vi "MC AOTF Engine.vi"(0 "Notifier Name":string, 11 "Ports (Unused)":string[](array[string])) -> ()   [LabVIEW 2016]
uses:
  AOTF Controls/AOTF Notifier Element.ctl
  AOTF Controls/AOTF Actions.ctl
  AOTF Controls/AOTF Lines Lines Control.ctl
  <vilib>/ULx/Create Channel.llb/ULx Create Channel (DO-Digital Output).vi
  <vilib>/ULx/Write.llb/ULx Write (Digital Bool 1Line 1Point).vi
  <vilib>/ULx/Create Channel.llb/ULx Create Channel (AO-Voltage-Basic).vi
  <vilib>/ULx/Write.llb/ULx Write (Analog 1D DBL 1Chan 1Samp).vi
panel:
  in  "Blank":bool
  in  "Quit":bool
  in  "546":dbl(slide) scale=0.0..100.0
  in  "642":dbl(slide) scale=0.0..100.0
  in  "560":dbl(slide) scale=0.0..100.0
  in  "488":dbl(slide) scale=0.0..100.0
  in  "405":dbl(slide) scale=0.0..100.0
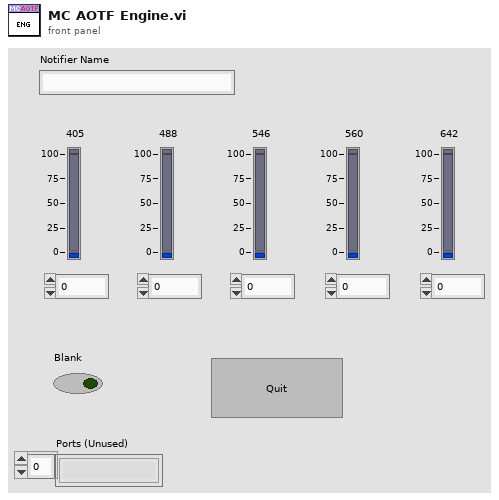
[diagram p1: front panel]
types:
  T1 = typedef "AOTF Lines Lines Control.ctl" = cluster{"Wavelength":u16[], "AO Line":string[]}
  T2 = typedef "AOTF Notifier Element.ctl" = cluster{"AOTF Action":T3, "Laser Line":string, "Power (%)":dbl, "Beam Blank On/Off":bool, "Line On/Off":bool, "Error":errorcluster}
  T3 = typedef "AOTF Actions.ctl" = enum16{"Error Check", "Blank", "Line On/Off", "Set Power", "Status", "Quit"}
  T4 = enum32{"Invalid", "Standard", "Closed", "Hidden", "Minimized", "Maximized"}
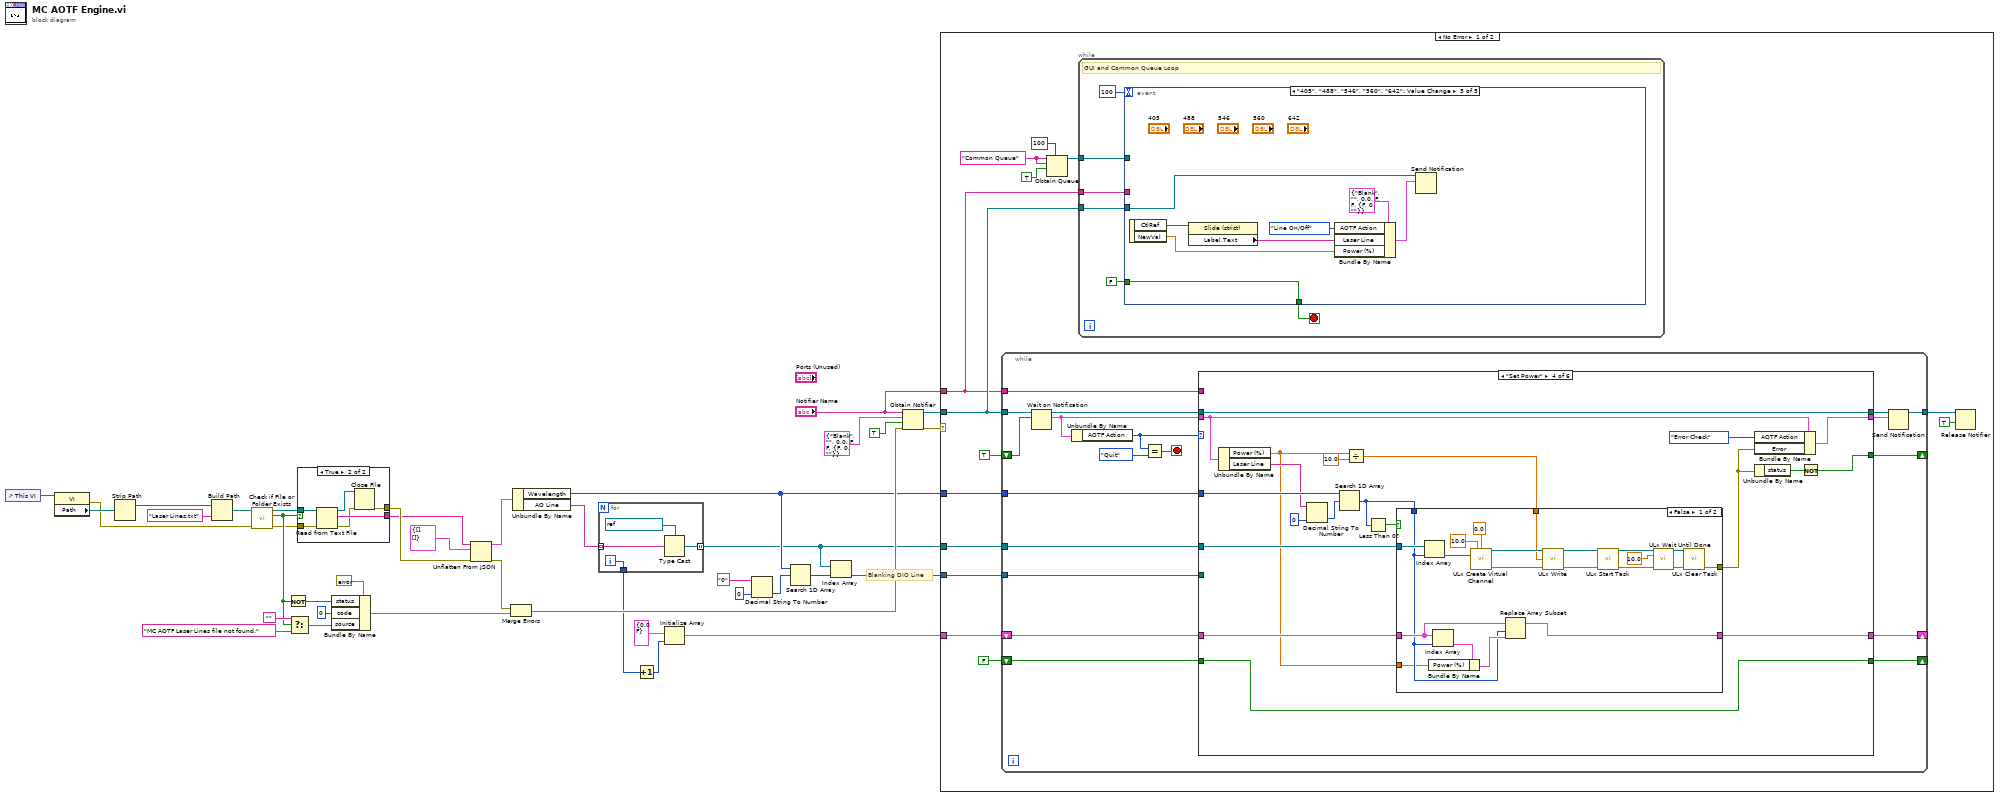
[diagram p0: block diagram]
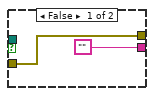
[diagram p2: hidden frame]
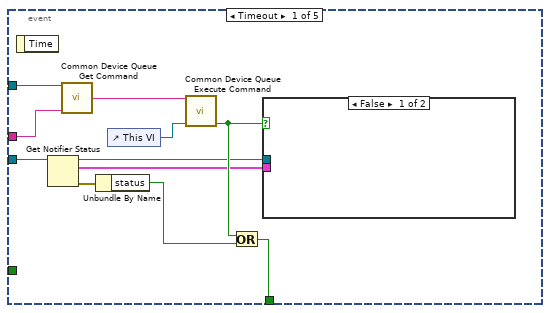
[diagram p3: hidden frame]
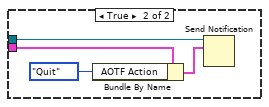
[diagram p4: hidden frame]
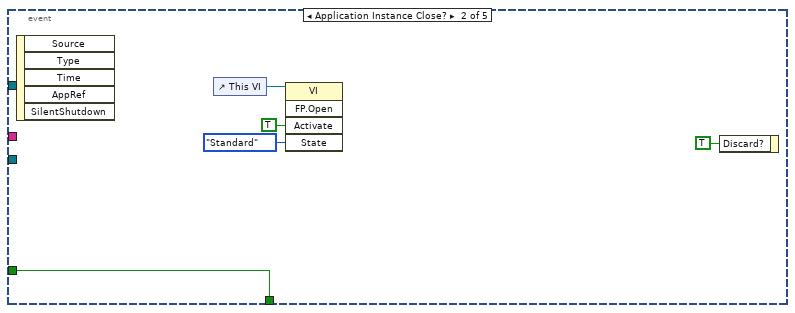
[diagram p5: hidden frame]
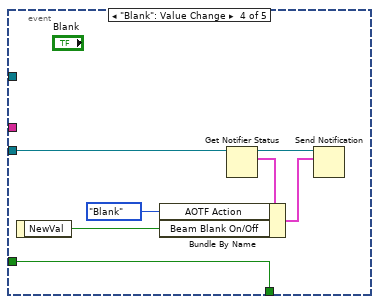
[diagram p6: hidden frame]
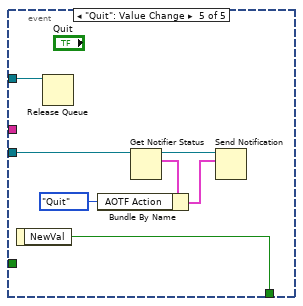
[diagram p7: hidden frame]
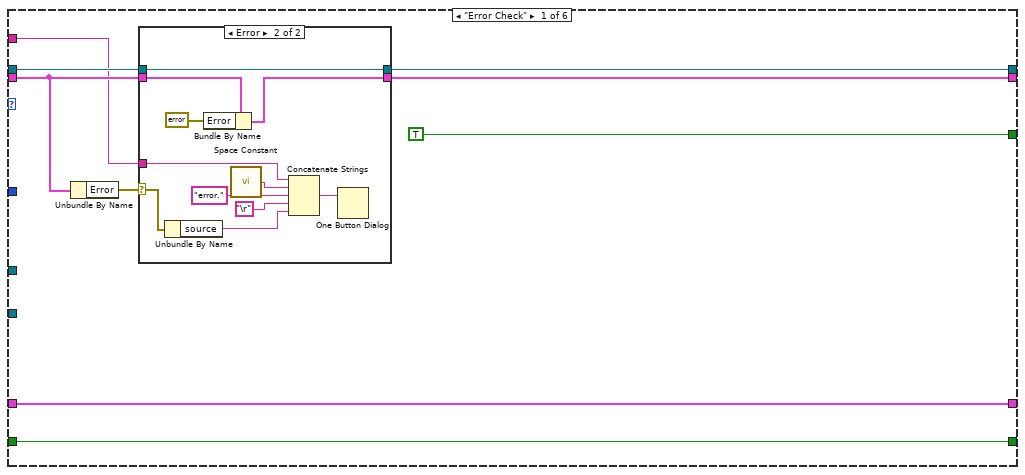
[diagram p8: hidden frame]
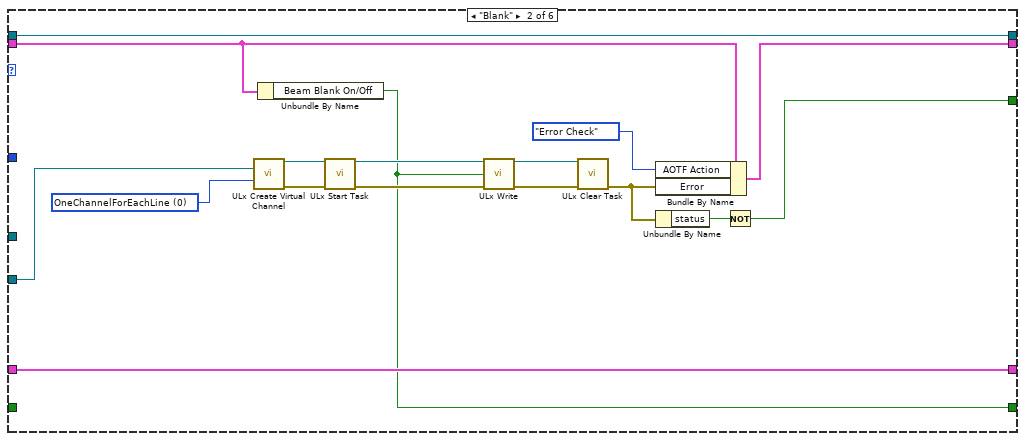
[diagram p10: hidden frame]
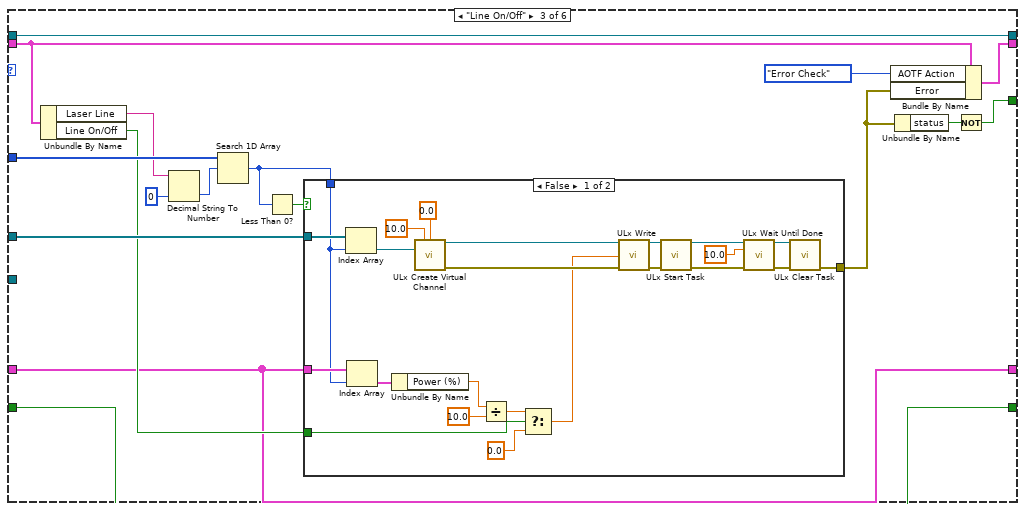
[diagram p11: hidden frame]
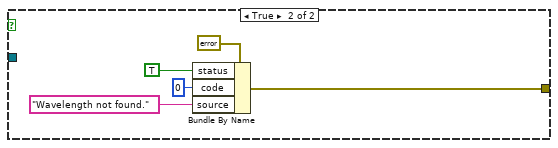
[diagram p12: hidden frame]
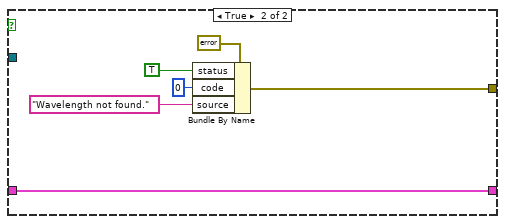
[diagram p13: hidden frame]
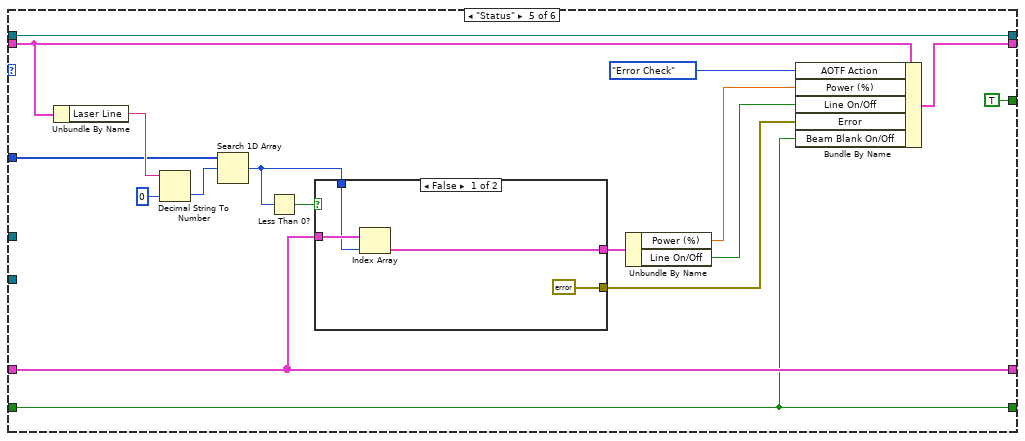
[diagram p14: hidden frame]
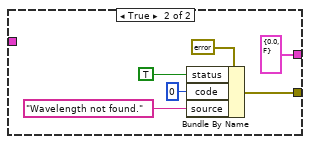
[diagram p15: hidden frame]
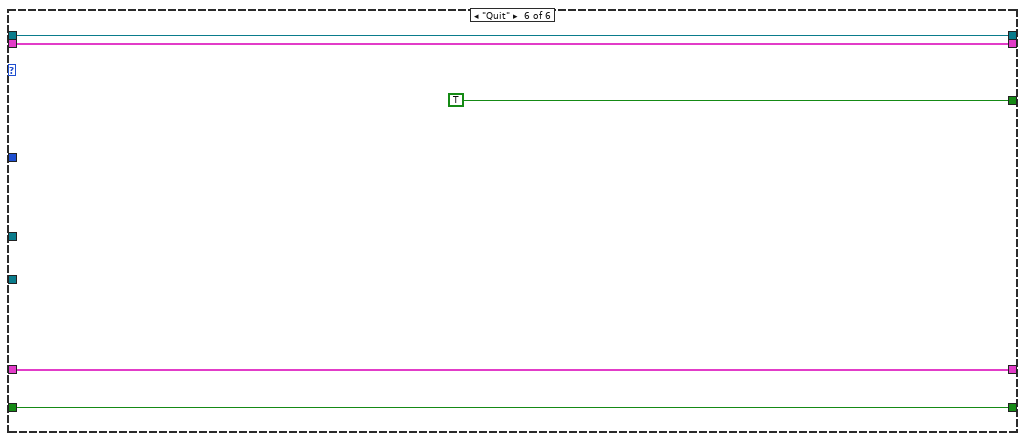
[diagram p16: hidden frame]
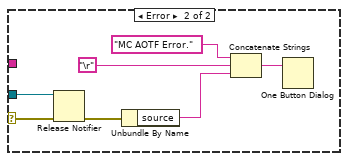
[diagram p17: hidden frame]
diagram:
  # "Blanking DIO Line"
  n1 = control-ref of="This VI"() -> (w37:refnum<vi>)
  n2 = property class="VI"(reference=w37) -> (error out=w21:errorcluster, "Path"=w36:path)  [unwired: 1 in, 1 out]
  n3 = Strip Path(path=w36) -> (stripped path=w35:path)  [unwired: 1 out]
  n4 = Build Path(base path=w35, name or relative path="Laser Lines.txt") -> (appended path=w33:path)
  n5 = call <vilib>:"Check if File or Folder Exists.vi"("error in (no error)"=w21, "path"=w33) -> ("error out"=w20:errorcluster, "file or folder exists?"=w23:bool, "dup path"=w22:path)  [unwired: 7 in]
  n6 = Not(x=w23) -> (.not. x?=w28:bool)
  n7 = Select(t="", s=w23, f="MC AOTF Laser Lines file not found." ("source")) -> (s? t:f=w24:string)
  n8 = case shown="True" w23 {
    tunnel: w22 -> [_ w47]
    tunnel: ["" w46] -> w15
    tunnel: w20 -> [w40 w44]
    tunnel: [w40 w42] -> w19
    frame False {
    }
    frame True {
      n9 = Read from Text File(file (use dialog)=w47, error in=w44) -> (refnum out=w45:refnum<file>, text=w46:string, error out=w43:errorcluster)  [unwired: 2 in, 1 out]
      n10 = Close File(refnum=w45, error in=w43) -> (error out=w42:errorcluster)  [unwired: 1 out]
    }
  }
  n11 = Bundle By Name(cluster=errorcluster {"status"=FALSE, "code"=0, "source"=""} ("Error"), "status"=w28, "code"=0, "source"=w24) -> (w17:errorcluster)
  n12 = Unflatten From JSON(JSON string=w15, type and defaults=T1 {"Wavelength"=[], "AO Line"=[]} ("Laser Lines"), error in (no error)=w19) -> (value=w13:T1, error out=w18:errorcluster)  [unwired: 4 in]
  n13 = Merge Errors(w18, w17) -> (w16:errorcluster)
  n14 = Unbundle By Name(w13) -> ("Wavelength"=w10:u16[], "AO Line"=w12:string[])
  n15 = for {
    tunnel: w12 -> [w50] mode=indexing
    tunnel: [w49] -> w7 mode=indexing
    tunnel: [w48] -> w2
    i -> [w48]
    n16 = Type Cast(type=refnum<k21> "Dev0/Ao12" ("Type Thingy"), x=w50) -> (*(type *) &x=w49:refnum<k21>)
  }
  n17 = Increment(x=w2) -> (x+1=w3:i32)
  n18 = Initialize Array(cluster{"Power (%)":dbl, "Line On/Off":bool} {"Power (%)"=0.0, "Line On/Off"=FALSE} ("Line Staus Cluster"), w3) -> (w1:cluster{"Power (%)":dbl, "Line On/Off":bool}[])
  n19 = Decimal String To Number(string="0", default (0L)=u16 0 ("default (0 I32)")) -> (number=w8:u16)  [unwired: 1 in, 1 out]
  n20 = Search 1D Array(1D array=w10, element=w8) -> (index of element=w6:i32)  [unwired: 1 in]
  n21 = Index Array(array=w7, index=w6) -> (element=w5:refnum<k21>)
  n22 = Obtain Notifier(name (unnamed)="Notifier Name", notification data type=T2 {"AOTF Action"=enum."Blank", "Laser Line"="", "Power (%)"=0.0, "Beam Blank On/Off"=FALSE, "Line On/Off"=FALSE, "Error"={"status"=FALSE, "code"=0, "source"=""}} ("AOTFQueueCtrl"), create if not found? (T)=TRUE, error in (no error)=w16) -> (notifier out=w32:refnum<notifier>, error out=w31:errorcluster)  [unwired: 1 out]
  n23 = case shown="No Error" w31 {
    selector: w31 -> [_ w301]
    tunnel: w32 -> [w61 w302]
    tunnel: "Notifier Name" -> [w57 _]
    tunnel: w10 -> [w56 _]
    tunnel: w7 -> [w55 _]
    tunnel: w5 -> [w54 _]
    tunnel: w1 -> [w52 _]
    frame No Error {
      w65 = "Common Queue" ("Unique Notifier Name")
      n24 = while {
        tunnel: w61 -> [w132]
        shift-right: [w123] -> _
        shift-left: TRUE ("ignore previous (F)") -> [w131]
        tunnel: [w122] -> w59
        tunnel: w57 -> [w121]
        tunnel: w56 -> [w120]
        tunnel: w55 -> [w119]
        tunnel: w54 -> [w118]
        shift-right: [w114] -> _
        shift-left: FALSE -> [w115]
        shift-right: [w116] -> _
        shift-left: w52 -> [w117]
        stop <- w126 stop-if-true
        n25 = Wait on Notification(notifier=w132, ignore previous (F)=w131) -> (notifier out=w130:refnum<notifier>, notification=w129:T2)  [unwired: 2 in, 2 out]
        n26 = Unbundle By Name(w129) -> ("AOTF Action"=w128:T3)
        n27 = Equal?(x=w128, y=AOTF_Actions."Quit") -> (x = y?=w126:bool)
        n28 = case shown="\"Set Power\"" w128 {
          tunnel: w130 -> [w141 w164 w186 w234 w280 w295]
          tunnel: w129 -> [w139 w163 w179 w225 w266 w294]
          tunnel: [w137 w164 w186 w234 w280 w295] -> w125
          tunnel: [w136 w162 w178 w224 w268 w294] -> w124
          tunnel: [TRUE w158 w177 w223 TRUE TRUE] -> w123
          tunnel: w121 -> [w138 _ _ _ _ _]
          tunnel: w120 -> [_ _ w188 w236 w269 _]
          tunnel: w119 -> [_ _ w187 w235 _ _]
          tunnel: w118 -> [_ w157 _ _ _ _]
          tunnel: w117 -> [w134 w156 w172 w220 w265 w292]
          tunnel: [w134 w156 w172 w219 w265 w292] -> w116
          tunnel: w115 -> [w133 _ w173 w218 w264 w291]
          tunnel: [w133 w155 w173 w218 w264 w291] -> w114
          frame "Error Check" {
            n29 = Unbundle By Name(w139) -> ("Error"=w140:errorcluster)
            n30 = case shown="Error" w140 {
              selector: w140 -> [_ w147]
              tunnel: w139 -> [w142 w151]
              tunnel: [w143 w149] -> w137
              tunnel: w141 -> [w143 w149]
              tunnel: w138 -> [_ w146]
              tunnel: [w142 w148] -> w136
              frame No Error {
              }
              frame Error {
                n31 = Unbundle By Name(w147) -> ("source"=w145:string)
                n32 = Bundle By Name(cluster=w151, "Error"=errorcluster {"status"=FALSE, "code"=0, "source"=""}) -> (w148:T2)
                n33 = call <vilib>:"Space Constant.vi"() -> ("String"=w154:string)
                n34 = Concatenate Strings(w146, w154, "error." ("string"), "\r", w145) -> (w152:string)
                n35 = One Button Dialog(message=w152) -> ()  [unwired: 1 in, 1 out]
              }
            }
          }
          frame "Blank" {
            w165 = 0 items=["OneChannelForEachLine", "OneChannelForAllLines"] ("line grouping")
            n36 = call-poly <vilib>:"ULx Create Virtual Channel.vi"("lines"=w157, "line grouping"=w165) -> ("task out"=w166:refnum<k24>, "error out"=w167:errorcluster)  [unwired: 12 in]
            n37 = Unbundle By Name(w163) -> ("Beam Blank On/Off"=w155:bool)
            n38 = call <vilib>:"ULx Start Task.vi"("task in"=w166, "error in"=w167) -> ("task out"=w168:refnum<k24>, "error out"=w169:errorcluster)  [unwired: 12 in]
            n39 = call-poly <vilib>:"ULx Write.vi"("task in"=w168, "data"=w155, "error in"=w169) -> ("task out"=w170:refnum<k24>, "error out"=w171:errorcluster)  [unwired: 10 in, 1 out]
            n40 = call <vilib>:"ULx Clear Task.vi"("task in"=w170, "error in"=w171) -> ("error out"=w160:errorcluster)  [unwired: 13 in]
            n41 = Bundle By Name(cluster=w163, "AOTF Action"=AOTF_Actions."Error Check", "Error"=w160) -> (w162:T2)
            n42 = Unbundle By Name(w160) -> ("status"=w159:bool)
            n43 = Not(x=w159) -> (.not. x?=w158:bool)
          }
          frame "Line On/Off" {
            n44 = Unbundle By Name(w179) -> ("Laser Line"=w185:string, "Line On/Off"=w174:bool)
            n45 = Decimal String To Number(string=w185, default (0L)=u16 0 ("default (0 I32)")) -> (number=w183:u16)  [unwired: 1 in, 1 out]
            n46 = Search 1D Array(1D array=w188, element=w183) -> (index of element=w175:i32)  [unwired: 1 in]
            n47 = Less Than 0?(x=w175) -> (x < 0?=w176:bool)
            n48 = case shown="False" w176 {
              tunnel: w187 -> [w211 _]
              tunnel: [w199 w212] -> w180
              tunnel: w175 -> [w196 _]
              tunnel: w172 -> [w197 _]
              tunnel: w174 -> [w190 _]
              frame False {
                n49 = Index Array(array=w211, index=w196) -> (element=w200:refnum<k21>)
                n50 = Index Array(array=w197, index=w196) -> (element=w195:cluster{"Power (%)":dbl, "Line On/Off":bool})
                n51 = Unbundle By Name(w195) -> ("Power (%)"=w192:dbl)
                n52 = call-poly <vilib>:"ULx Create Virtual Channel.vi"("maximum value"=10.0, "minimum value"=0.0, "physical channels"=w200) -> ("task out"=w210:refnum<k24>, "error out"=w203:errorcluster)  [unwired: 11 in]
                n53 = Divide(x=w192, y=10.0) -> (x/y=w191:dbl)
                n54 = Select(t=w191, s=w190, f=0.0 ("minimum value")) -> (s? t:f=w189:dbl)
                n55 = call-poly <vilib>:"ULx Write.vi"("task in"=w210, "data"=w189, "error in"=w203) -> ("task out"=w198:refnum<k24>, "error out"=w204:errorcluster)  [unwired: 10 in, 1 out]
                n56 = call <vilib>:"ULx Start Task.vi"("task in"=w198, "error in"=w204) -> ("task out"=w209:refnum<k24>, "error out"=w206:errorcluster)  [unwired: 12 in]
                n57 = call <vilib>:"ULx Wait Until Done.vi"("task in"=w209, "timeout"=10.0, "error in"=w206) -> ("task out"=w208:refnum<k24>, "error out"=w205:errorcluster)  [unwired: 11 in]
                n58 = call <vilib>:"ULx Clear Task.vi"("task in"=w208, "error in"=w205) -> ("error out"=w199:errorcluster)  [unwired: 13 in]
              }
              frame True {
                n59 = Bundle By Name(cluster=errorcluster {"status"=FALSE, "code"=0, "source"=""} ("error out"), "status"=TRUE, "code"=0, "source"="Wavelength not found.") -> (w212:errorcluster)
              }
            }
            n60 = Bundle By Name(cluster=w179, "AOTF Action"=AOTF_Actions."Error Check", "Error"=w180) -> (w178:T2)
            n61 = Unbundle By Name(w180) -> ("status"=w181:bool)
            n62 = Not(x=w181) -> (.not. x?=w177:bool)
          }
          frame "Set Power" {
            n63 = Unbundle By Name(w225) -> ("Power (%)"=w217:dbl, "Laser Line"=w233:string)
            n64 = Decimal String To Number(string=w233, default (0L)=u16 0 ("default (0 I32)")) -> (number=w231:u16)  [unwired: 1 in, 1 out]
            n65 = Search 1D Array(1D array=w236, element=w231) -> (index of element=w221:i32)  [unwired: 1 in]
            n66 = Divide(x=w217, y=10.0) -> (x/y=w229:dbl)
            n67 = Less Than 0?(x=w221) -> (x < 0?=w222:bool)
            n68 = case shown="False" w222 {
              tunnel: w235 -> [w257 _]
              tunnel: w229 -> [w245 _]
              tunnel: [w244 w259] -> w226
              tunnel: w221 -> [w239 _]
              tunnel: w220 -> [w240 w258]
              tunnel: [w238 w258] -> w219
              tunnel: w217 -> [w237 _]
              frame False {
                n69 = Index Array(array=w257, index=w239) -> (element=w246:refnum<k21>)
                n70 = Index Array(array=w240, index=w239) -> (element=w242:cluster{"Power (%)":dbl, "Line On/Off":bool})
                n71 = Bundle By Name(cluster=w242, "Power (%)"=w237) -> (w241:cluster{"Power (%)":dbl, "Line On/Off":bool})
                n72 = call-poly <vilib>:"ULx Create Virtual Channel.vi"("maximum value"=10.0, "minimum value"=0.0, "physical channels"=w246) -> ("task out"=w256:refnum<k24>, "error out"=w249:errorcluster)  [unwired: 11 in]
                n73 = Replace Array Subset(array=w240, new element=w241, index=w239) -> (w238:cluster{"Power (%)":dbl, "Line On/Off":bool}[])
                n74 = call-poly <vilib>:"ULx Write.vi"("task in"=w256, "data"=w245, "error in"=w249) -> ("task out"=w243:refnum<k24>, "error out"=w250:errorcluster)  [unwired: 10 in, 1 out]
                n75 = call <vilib>:"ULx Start Task.vi"("task in"=w243, "error in"=w250) -> ("task out"=w255:refnum<k24>, "error out"=w252:errorcluster)  [unwired: 12 in]
                n76 = call <vilib>:"ULx Wait Until Done.vi"("task in"=w255, "timeout"=10.0, "error in"=w252) -> ("task out"=w254:refnum<k24>, "error out"=w251:errorcluster)  [unwired: 11 in]
                n77 = call <vilib>:"ULx Clear Task.vi"("task in"=w254, "error in"=w251) -> ("error out"=w244:errorcluster)  [unwired: 13 in]
              }
              frame True {
                n78 = Bundle By Name(cluster=errorcluster {"status"=FALSE, "code"=0, "source"=""} ("error out"), "status"=TRUE, "code"=0, "source"="Wavelength not found.") -> (w259:errorcluster)
              }
            }
            n79 = Bundle By Name(cluster=w225, "AOTF Action"=AOTF_Actions."Error Check", "Error"=w226) -> (w224:T2)
            n80 = Unbundle By Name(w226) -> ("status"=w227:bool)
            n81 = Not(x=w227) -> (.not. x?=w223:bool)
          }
          frame "Status" {
            n82 = Unbundle By Name(w266) -> ("Laser Line"=w272:string)
            n83 = Decimal String To Number(string=w272, default (0L)=u16 0 ("default (0 I32)")) -> (number=w271:u16)  [unwired: 1 in, 1 out]
            n84 = Search 1D Array(1D array=w269, element=w271) -> (index of element=w274:i32)  [unwired: 1 in]
            n85 = Less Than 0?(x=w274) -> (x < 0?=w273:bool)
            n86 = case shown="False" w273 {
              tunnel: w265 -> [w284 _]
              tunnel: [errorcluster {"status"=FALSE, "code"=0, "source"=""} ("error out") w286] -> w276
              tunnel: w274 -> [w283 _]
              tunnel: [w282 cluster{"Power (%)":dbl, "Line On/Off":bool} {"Power (%)"=0.0, "Line On/Off"=FALSE} ("Line Staus Cluster")] -> w277
              frame False {
                n87 = Index Array(array=w284, index=w283) -> (element=w282:cluster{"Power (%)":dbl, "Line On/Off":bool})
              }
              frame True {
                n88 = Bundle By Name(cluster=errorcluster {"status"=FALSE, "code"=0, "source"=""} ("error out"), "status"=TRUE, "code"=0, "source"="Wavelength not found.") -> (w286:errorcluster)
              }
            }
            n89 = Unbundle By Name(w277) -> ("Power (%)"=w278:dbl, "Line On/Off"=w279:bool)
            n90 = Bundle By Name(cluster=w266, "AOTF Action"=AOTF_Actions."Error Check", "Power (%)"=w278, "Line On/Off"=w279, "Error"=w276, "Beam Blank On/Off"=w264) -> (w268:T2)
          }
          frame "Quit" {
          }
        }
        n91 = Send Notification(notification=w124, notifier=w125) -> (notifier out=w122:refnum<notifier>)  [unwired: 1 in, 1 out]
      }
      n92 = Obtain Queue(max queue size (-1, unlimited)=100, name (unnamed)=w65, element data type=w65, create if not found? (T)=TRUE) -> (queue out=w62:refnum<queue>)  [unwired: 1 in, 2 out]
      n93 = while {
        tunnel: w62 -> [w70]
        tunnel: w57 -> [w68]
        tunnel: w61 -> [w69]
        stop <- w67 stop-if-true
        # "GUI and Common Queue Loop"
        n94 = event shown="[2] \"405\", \"488\", \"546\", \"560\", \"642\": Value Change" {
          selector: _ -> [_ _ _ _ _]
          dyn-events: _ -> [_ _ _ _ _]
          timeout: 100 -> [_ _ _ _ _]
          tunnel: w70 -> [w77 _ _ _ w113]
          tunnel: w69 -> [w73 _ w98 w105 w112]
          tunnel: w68 -> [w76 _ _ _ _]
          tunnel: [w75 w91 w99 w106 w110] -> w67
          tunnel: FALSE -> [_ w91 w99 w106 _]
          event Timeout {
            n95 = event-data() -> ()  [unwired: 1 in, 1 out]
            n96 = Get Notifier Status(notifier=w73) -> (notifier out=w72:refnum<notifier>, current notification=w74:T2, error out=w82:errorcluster)  [unwired: 1 in, 2 out]
            n97 = call "Common Device Queue Get Command.vi"("Common Queue"=w77, "Notifier Name"=w76) -> ("Command"=w81:string)  [unwired: 12 in, 1 out]
            n98 = Unbundle By Name(w82) -> ("status"=w79:bool)
            n99 = control-ref of="This VI"() -> (w80:refnum<vi>)
            n100 = call "Common Device Queue Execute Command.vi"("Common Command"=w81, "VI Refnum"=w80) -> ("Quit?"=w78:bool)  [unwired: 12 in, 1 out]
            n101 = Or(x=w78, y=w79) -> (x .or. y?=w75:bool)
            n102 = case shown="False" w78 {
              tunnel: w72 -> [_ w86]
              tunnel: w74 -> [_ w85]
              frame False {
              }
              frame True {
                n103 = Bundle By Name(cluster=w85, "AOTF Action"=AOTF_Actions."Quit") -> (w84:T2)
                n104 = Send Notification(notification=w84, notifier=w86) -> ()  [unwired: 1 in, 2 out]
              }
            }
          }
          event Application Instance Close? {
            n105 = event-data() -> ()  [unwired: 1 in, 5 out]
            n106 = control-ref of="This VI"() -> (w88:refnum<vi>)
            n107 = invoke class="VI" method="FP.Open"(reference=w88, "Activate"=TRUE ("Activate?"), "State"=T4."Standard") -> ()  [unwired: 2 in, 5 out]
            n108 = event-data("Discard?"=TRUE) -> ()  [unwired: 1 in, 1 out]
          }
          event "405", "488", "546", "560", "642": Value Change {
            n109 = event-data() -> ("CtlRef"=w97:refnum<vi>, "NewVal"=w93:dbl)  [unwired: 1 in]
            n110 = property class="Slide (strict)"(reference=w97) -> ("Label.Text"=w94:string)  [unwired: 1 in, 2 out]
            n111 = Bundle By Name(cluster=T2 {"AOTF Action"=enum."Blank", "Laser Line"="", "Power (%)"=0.0, "Beam Blank On/Off"=FALSE, "Line On/Off"=FALSE, "Error"={"status"=FALSE, "code"=0, "source"=""}} ("AOTFQueueCtrl"), "AOTF Action"=AOTF_Actions."Line On/Off", "Laser Line"=w94, "Power (%)"=w93) -> (w92:T2)
            n112 = Send Notification(notification=w92, notifier=w98) -> ()  [unwired: 1 in, 2 out]
          }
          event "Blank": Value Change {
            n113 = event-data() -> ("NewVal"=w101:bool)  [unwired: 1 in]
            n114 = Get Notifier Status(notifier=w105) -> (notifier out=w104:refnum<notifier>, current notification=w103:T2)  [unwired: 1 in, 3 out]
            n115 = Bundle By Name(cluster=w103, "AOTF Action"=AOTF_Actions."Blank", "Beam Blank On/Off"=w101) -> (w100:T2)
            n116 = Send Notification(notification=w100, notifier=w104) -> ()  [unwired: 1 in, 2 out]
          }
          event "Quit": Value Change {
            n117 = event-data() -> ("NewVal"=w110:bool)  [unwired: 1 in]
            n118 = Release Queue(queue=w113) -> ()  [unwired: 2 in, 3 out]
            n119 = Get Notifier Status(notifier=w112) -> (notifier out=w111:refnum<notifier>, current notification=w109:T2)  [unwired: 1 in, 3 out]
            n120 = Bundle By Name(cluster=w109, "AOTF Action"=AOTF_Actions."Quit") -> (w107:T2)
            n121 = Send Notification(notification=w107, notifier=w111) -> ()  [unwired: 1 in, 2 out]
          }
        }
      }
      n122 = Release Notifier(notifier=w59, force destroy? (F)=TRUE) -> ()  [unwired: 1 in, 3 out]
    }
    frame Error {
      n123 = Release Notifier(notifier=w302, error in (no error)=w301) -> (error out=w298:errorcluster)  [unwired: 1 in, 2 out]
      n124 = Unbundle By Name(w298) -> ("source"=w297:string)
      n125 = Concatenate Strings("MC AOTF Error.", "\r", w297) -> (w296:string)
      n126 = One Button Dialog(message=w296) -> ()  [unwired: 1 in, 1 out]
    }
  }
